vi "TopLevel.vi"   [LabVIEW 2021]
uses:
  <vilib>/Platform/TimedLoop/XDataNode/timing_clust.ctl
  <vilib>/Platform/TimedLoop/XDataNode/nitl_modes.ctl
  <vilib>/Platform/TimedLoop/XDataNode/wakeup.ctl
  <vilib>/rvi/Emulation/niFpgaSctlEmulationGetInTimedLoop.vi
  <vilib>/rvi/Emulation/niFpgaEmulationReportErrorSimple.vi
  <vilib>/rvi/Emulation/niFpgaGetClockAttributes.vi
  <vilib>/rvi/Emulation/niFpgaCriticalErrorInLSC.vi
  <vilib>/rvi/eio/common/nirviEmuTemplatePropertySet_noerrors.vi
  <vilib>/platform/TimedLoop/XDataNode/XDataNode.xnode
  <vilib>/eio/EIOPropertyNode/EIOPropertyNode.xnode
  <vilib>/Platform/TimedLoop/XDataNode/XDNodeRunTimeDep.lvlib
  <vilib>/rvi/eio/common/nirviEmuTemplatePropertyGet_errors.vi
  <vilib>/rvi/eio/common/nirviEmuTemplatePropertyGet_noerrors.vi
  <vilib>/rvi/eio/common/nirviEmuTemplatePropertySet_errors.vi
types:
  T1 = typedef "XDNodeRunTimeDep.lvlib/timing_clust.ctl" = cluster{"Expected End [f-1]":u64, "Actual End [f-1]":u64, "Finished Late? [f-1]":bool, "Expected End [i-1]":u64, "Actual End [i-1]":u64, "Finished Late? [i-1]":bool, "Expected Start [i]":u64, "Actual Start [i]":u64, "Expected Start [f]":u64, "Actual Start [f]":u64, "Source Name":string, "Structure Name":string, "Period":i64, "Deadline":i64, "Offset":i64, "Start":i64, "Priority":i32, "Timeout":i32, "Mode":T2, "Wakeup Reason":T3, "Error":errorcluster, "Source Type":string, "Secondary Source Type":string, "Global End Time":u64, "Global Start Time":u64, "Frame Duration":u64, "Iteration Duration":u64, "Assigned CPU":i32, "I/O Scan Engine Mode":u32}
  T2 = typedef "XDNodeRunTimeDep.lvlib/nitl_modes.ctl" = enum32{"No Change", "Process missed periods, maintain original phase", "Discard missed periods, maintain original phase", "Process missed periods, ignore original phase", "Discard missed periods, ignore original phase"}
  T3 = typedef "XDNodeRunTimeDep.lvlib/wakeup.ctl" = enum32{"Normal", "Aborted", "Asynchronous wakeup", "Timing source error", "Timed loop error", "Timeout"}
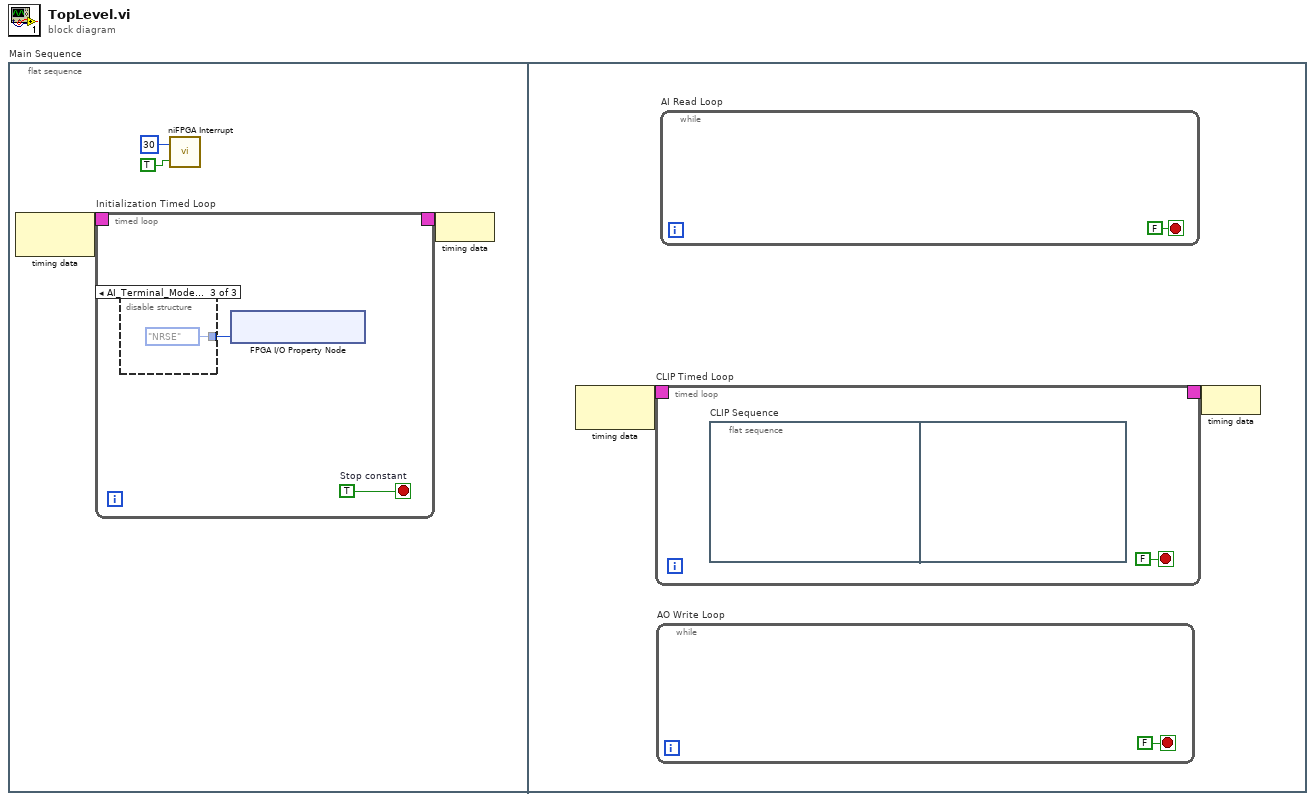
[diagram p0: block diagram]
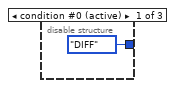
[diagram p2: hidden frame]
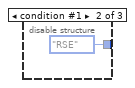
[diagram p3: hidden frame]
diagram:
  n1 = flat-sequence "Main Sequence" {
    frame #0 {
      n2 = node-c288 ("Input Node")() -> (w2:T1)  [unwired: 1 in]
      n3 = timed-loop "Initialization Timed Loop" {
        timing: w2 -> [_]
        timing-out: [_] -> w1
        stop <- w6 stop-if-true
        w6 = TRUE  # Stop constant
        n4 = disable-structure shown="AI_Terminal_Mode==NRSE" {
          disable-tunnel: [enum8{"DIFF", "RSE", "NRSE"}."DIFF" ("AI Terminal Mode") enum8{"DIFF", "RSE", "NRSE"}."RSE" ("AI Terminal Mode") enum8{"DIFF", "RSE", "NRSE"}."NRSE" ("AI Terminal Mode")] -> w5
          frame condition #0 (active) {
          }
          frame condition #1 {
          }
          frame condition #2 {
          }
        }
        n5 = xnode "FPGA I/O Property Node"("AI Terminal Mode"=w5) -> ()  [unwired: 1 in, 1 out]
      }
      n6 = call <vilib>:"niFPGA Interrupt.vi"("Wait Until Cleared (F)"=TRUE, "IRQ Number (0)"=u8 30) -> ()  [unwired: 1 in]
      n7 = node-c288 ("Output Node")(w1) -> ()
    }
    frame #1 {
      n8 = node-c288 ("Input Node")() -> (w15:T1)  [unwired: 1 in]
      n9 = timed-loop "CLIP Timed Loop" {
        timing: w15 -> [_]
        timing-out: [_] -> w14
        stop <- FALSE stop-if-true
        n10 = flat-sequence "CLIP Sequence" {
          frame #0 {
          }
          frame #1 {
          }
        }
      }
      n11 = while "AO Write Loop" {
        stop <- FALSE stop-if-true
      }
      n12 = while "AI Read Loop" {
        stop <- FALSE stop-if-true
      }
      n13 = node-c288 ("Output Node")(w14) -> ()
    }
  }
